vi "He magnet field realtime.vi"() -> ()   [LabVIEW 2016]
uses:
  <vilib>/rvi/interface/nirviReadWriteControl/nirviReadWriteControl.xnode
  <vilib>/rvi/interface/nirviOpenFPGA/nirviOpenFPGA.xnode
  HE Fpga/He magnet field fpga.vi
  <vilib>/Utility/error.llb/Error Cluster From Error Code.vi
  <vilib>/rvi/errors/niLvFpgaAdjustHostInterfaceError.vi
  NiFpgaLv.dll
  FPGA Bitfiles/Controlsoftware2_FPGATarget3_Hemagnetfieldfpg_5TwZ+QBV9Tk.lvbitx
  <vilib>/FPGAPlugInAG/cRIO-9074/niLvFpga_Open_cRIO-9074.vi
panel:
  out "He Quad B I":fxp<+/-,26,5> format="%.3g"
  in  "Ion gauge cluster control":T1
  in  "Tab Control":enum32{"Extra", "Controls"}(tab)
  out "Convectron 3":u8[](array[numeric])
  out "Ion gauge 4":u8[](array[numeric])
  out "Convectron 4":u8[](array[numeric])
  out "Ion gauge 5":u8[](array[numeric])
  out "Convectron 2":u8[](array[numeric])
  out "Ion gauge 2":u8[](array[numeric])
  out "Convectron 1":u8[](array[numeric])
  out "Ion gauge 1":u8[](array[numeric])
  out "He Quad B I":fxp<+/-,26,5> format="%.3g"
  out "He Quad B V":fxp<+/-,26,5> format="%.3g"
  out "He Quad A I":fxp<+/-,26,5> format="%.3g"
  out "He Quad A V":fxp<+/-,26,5> format="%.3g"
  out "Y-I":fxp<+/-,26,5> format="%.3g"
  out "Y-V":fxp<+/-,26,5> format="%.3g"
  out "Y+I":fxp<+/-,26,5> format="%.3g"
  out "Y+ V":fxp<+/-,26,5> format="%.3g"
  out "X-I":fxp<+/-,26,5> format="%.3g"
  out "X- V":fxp<+/-,26,5> format="%.3g"
  out "X+ I":fxp<+/-,26,5> format="%.3g"
  out "X+ V":fxp<+/-,26,5> format="%.3g"
  out "Y Steerer -":dbl
  out "Y Steerer +":dbl
  out "Y Steerer - 2":dbl
  out "Y Steerer + 2":dbl
  out "X Steerer -":dbl
  out "X Steerer +":dbl
  out "He Quad B":dbl
  out "He Quad A":dbl
  out "Y-I 2":fxp<+/-,26,5> format="%.3g"
  out "Y-V 2":fxp<+/-,26,5> format="%.3g"
  out "Y+I 2":fxp<+/-,26,5> format="%.3g"
  out "Y+ V  2":fxp<+/-,26,5> format="%.3g"
  out "Analyze IN?":bool
  out "Analyze Out?":bool
  out "Tank Exit FC":bool
  out "Analyze Image FC":bool
  out "Ion gauge cluser 2":T1
  out "Ion gauge Cluster 1":T1
  out "error out 3":errorcluster
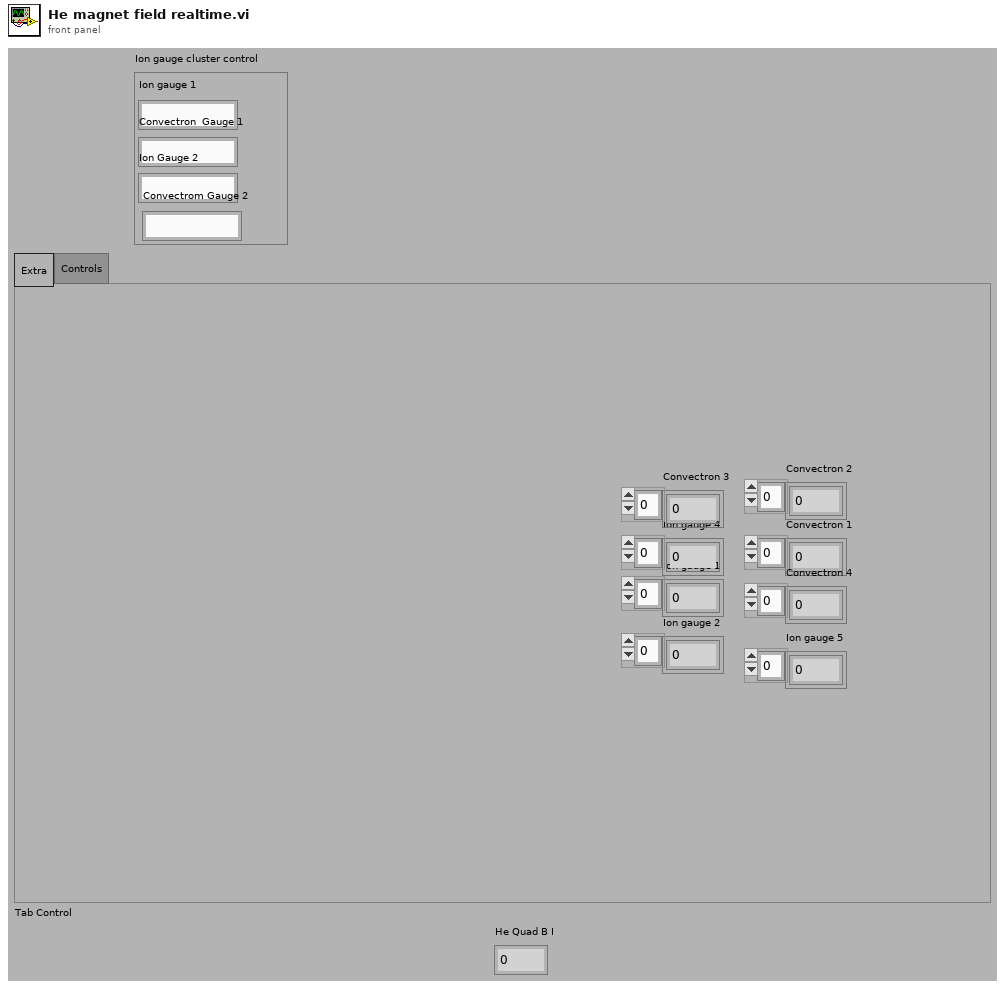
[diagram p1: front panel]
types:
  T1 = cluster{"Ion gauge 1":string, "Convectron  Gauge 1 ":string, "Ion Gauge 2":string, "Convectrom Gauge 2":string}
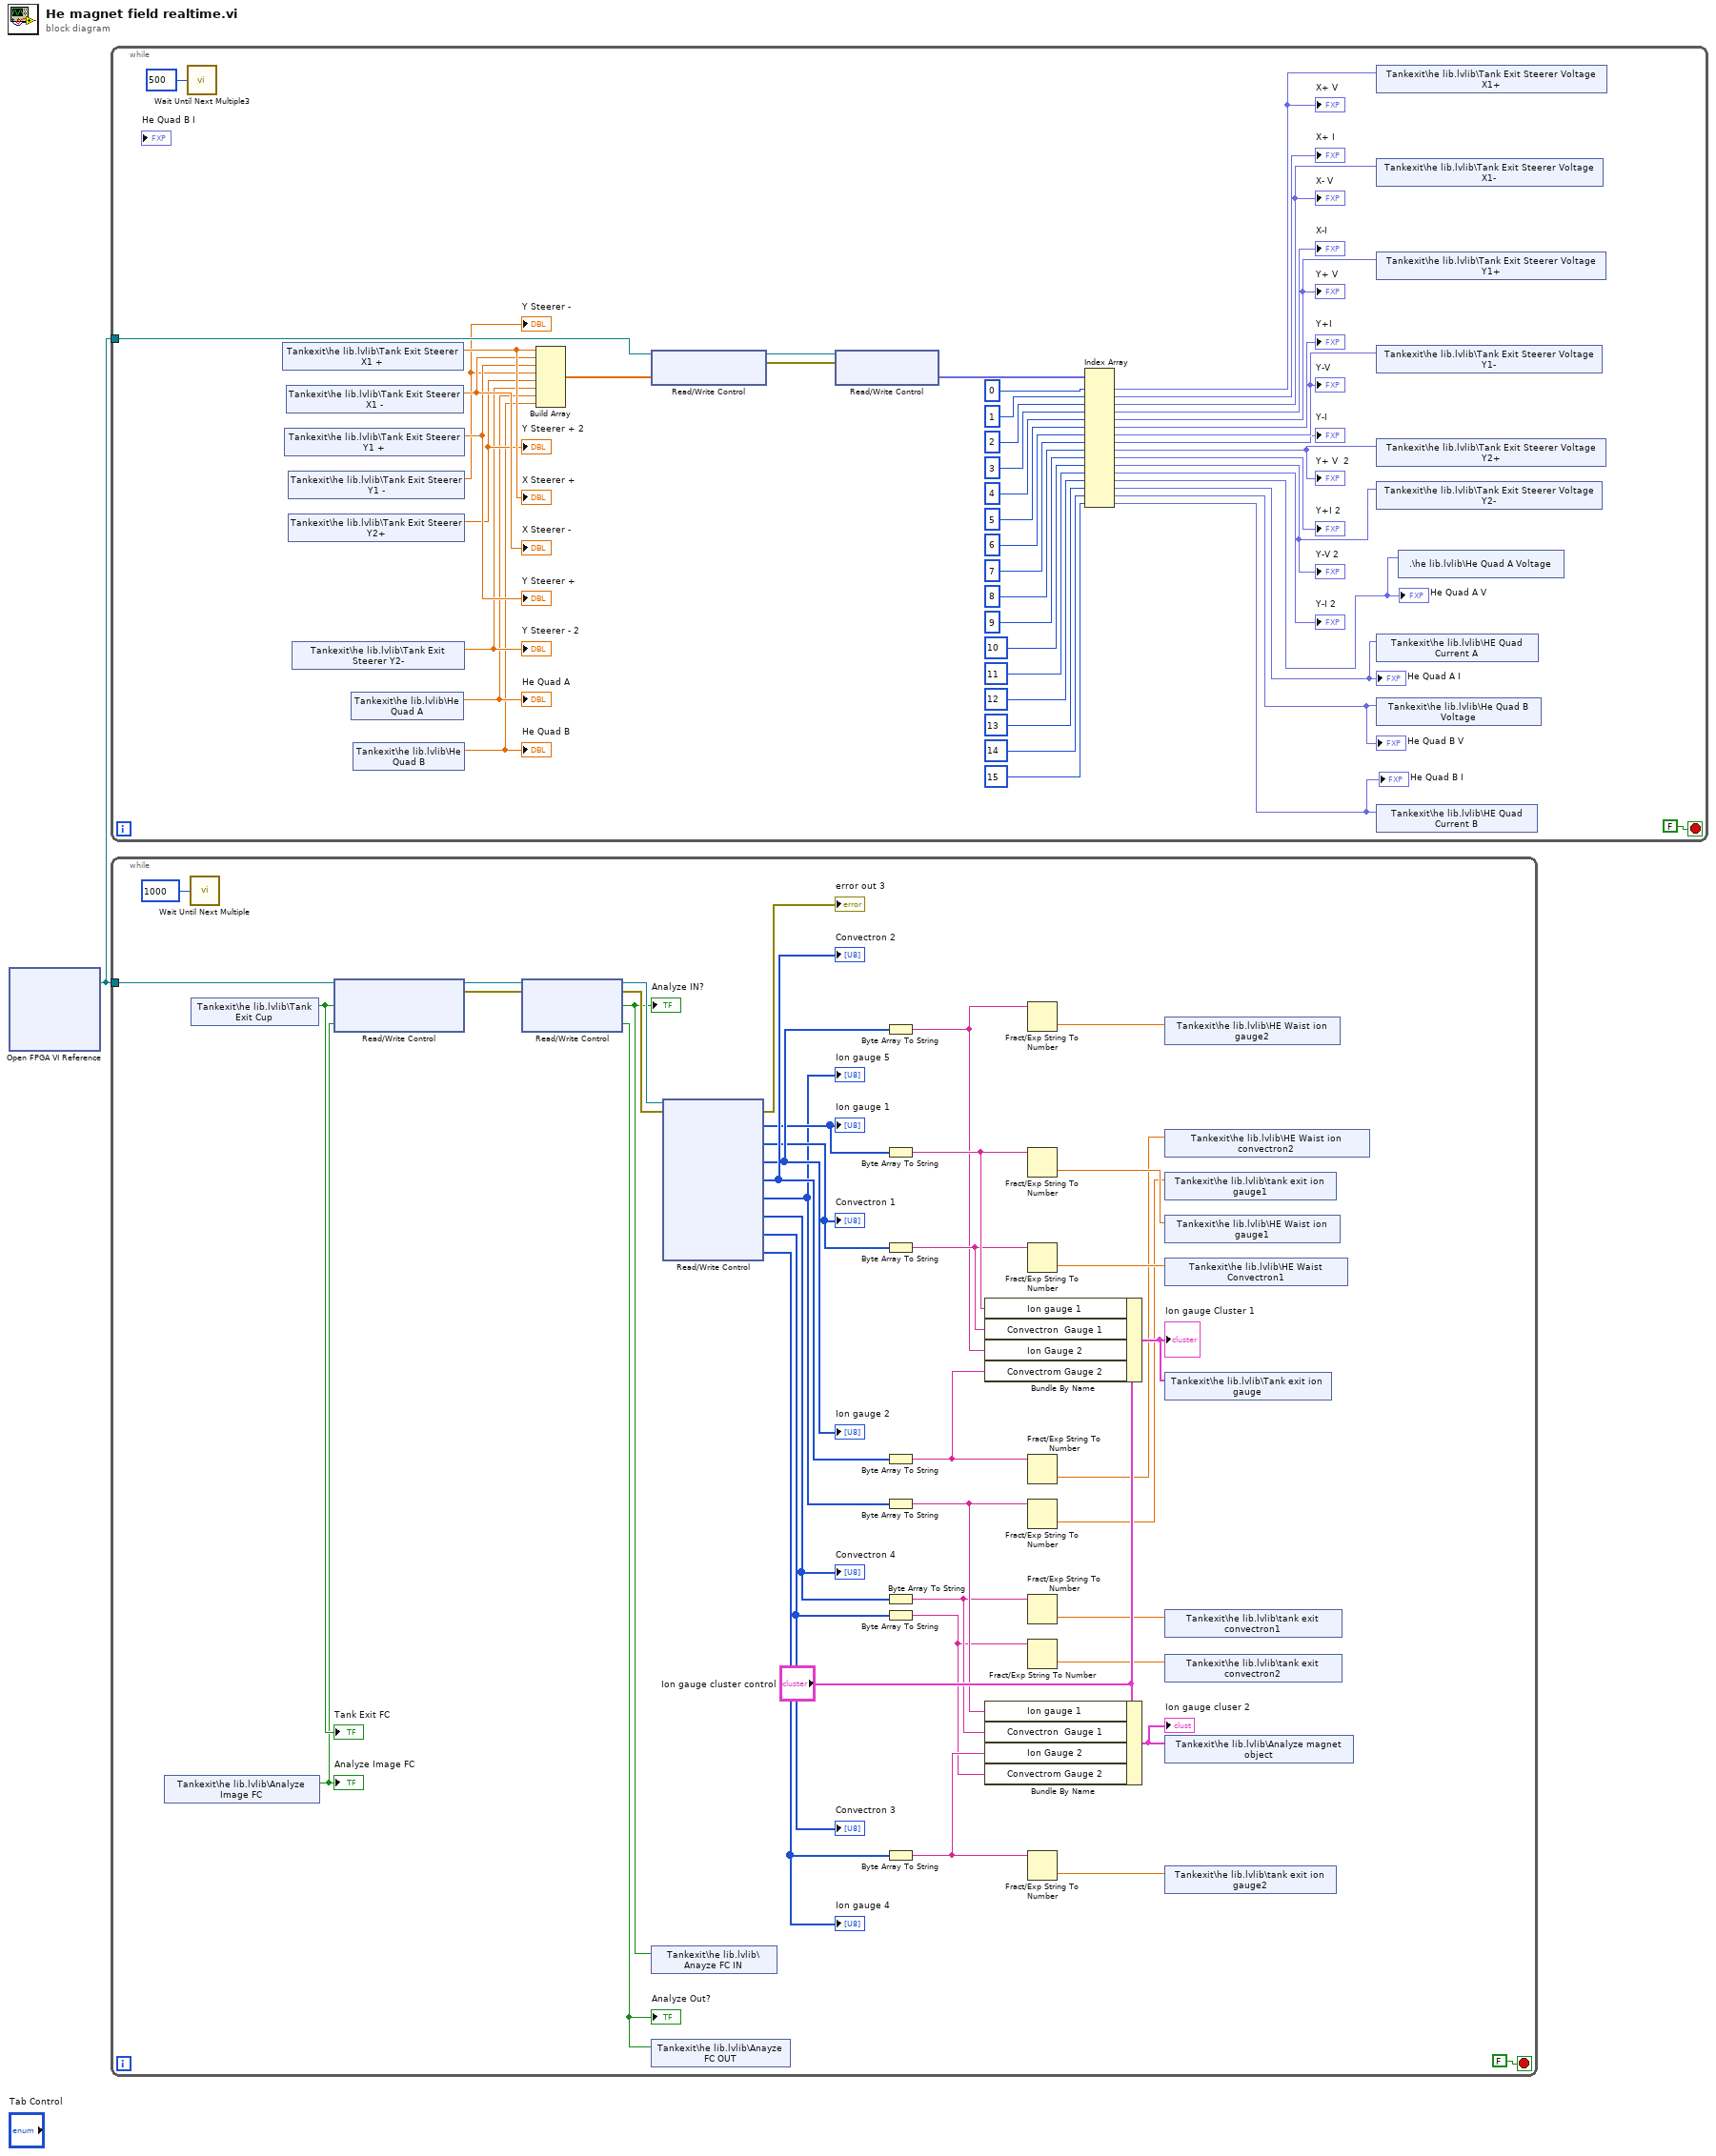
[diagram p0: block diagram]
diagram:
  n1 = xnode "Open FPGA VI Reference"() -> ("FPGA VI Reference Out"=w1:refnum<k20>)  [unwired: 2 in, 1 out]
  n2 = while {
    tunnel: w1 -> [w47]
    stop <- FALSE stop-if-true
    n3 = call "Wait Until Next Multiple3"("Count(mSec)"=u32 500 ("Count(uSec)")) -> ()  [unwired: 1 out]
    n4 = shared-variable "Tankexit\\he lib.lvlib\\Tank Exit Steerer X1 +"() -> (w25:dbl)  [unwired: 1 in, 1 out]
    "X Steerer +" <- w25
    n5 = shared-variable "Tankexit\\he lib.lvlib\\Tank Exit Steerer Y1 +"() -> (w23:dbl)  [unwired: 1 in, 1 out]
    "Y Steerer +" <- w23
    n6 = shared-variable "Tankexit\\he lib.lvlib\\Tank Exit Steerer X1 -"() -> (w24:dbl)  [unwired: 1 in, 1 out]
    "X Steerer -" <- w24
    n7 = shared-variable "Tankexit\\he lib.lvlib\\Tank Exit Steerer Y1 -"() -> (w22:dbl)  [unwired: 1 in, 1 out]
    "Y Steerer -" <- w22
    n8 = shared-variable "Tankexit\\he lib.lvlib\\Tank Exit Steerer Y2+"() -> (w21:dbl)  [unwired: 1 in, 1 out]
    "Y Steerer + 2" <- w21
    n9 = shared-variable "Tankexit\\he lib.lvlib\\Tank Exit Steerer Y2-"() -> (w20:dbl)  [unwired: 1 in, 1 out]
    "Y Steerer - 2" <- w20
    n10 = shared-variable "Tankexit\\he lib.lvlib\\He Quad A"() -> (w19:dbl)  [unwired: 1 in, 1 out]
    "He Quad A" <- w19
    n11 = shared-variable "Tankexit\\he lib.lvlib\\He Quad B"() -> (w18:dbl)  [unwired: 1 in, 1 out]
    "He Quad B" <- w18
    n12 = Build Array(w25, w24, w23, w22, w21, w20, w19, w18) -> (w48:dbl[])
    n13 = xnode "Read/Write Control"("FPGA VI Reference In"=w47, "Analog Output"=w48) -> ("FPGA VI Reference Out"=w34:refnum<k20>, "error out"=w30:errorcluster)  [unwired: 1 in]
    n14 = xnode "Read/Write Control"("FPGA VI Reference In"=w34, "error in"=w30) -> ("Analog input"=w33:fxp<+/-,26,5>[])  [unwired: 2 out]
    n15 = Index Array(array=w33, index #1=0 ("index"), index #2=1 ("index"), index #3=2 ("index"), index #4=3 ("index"), index #5=4 ("index"), index #6=5 ("index"), index #7=6 ("index"), index #8=7 ("index"), index #9=8 ("index"), index #10=9 ("index"), index #11=10 ("index"), index #12=11 ("index"), index #13=12 ("index"), index #14=13 ("index"), index #15=14 ("index"), index #16=15 ("index")) -> (element #1=w17:fxp<+/-,26,5>, element #2=→"X+ I":fxp<+/-,26,5>, element #3=w15:fxp<+/-,26,5>, element #4=→"X-I":fxp<+/-,26,5>, element #5=w13:fxp<+/-,26,5>, element #6=→"Y+I":fxp<+/-,26,5>, element #7=w11:fxp<+/-,26,5>, element #8=→"Y-I":fxp<+/-,26,5>, element #9=w9:fxp<+/-,26,5>, element #10=→"Y+I 2":fxp<+/-,26,5>, element #11=w6:fxp<+/-,26,5>, element #12=→"Y-I 2":fxp<+/-,26,5>, element #13=w3:fxp<+/-,26,5>, element #14=w4:fxp<+/-,26,5>, element #15=w5:fxp<+/-,26,5>, element #16=w2:fxp<+/-,26,5>)
    "X+ V" <- w17
    "X- V" <- w15
    "Y+ V" <- w13
    "Y-V" <- w11
    "He Quad A V" <- w3
    "He Quad A I" <- w4
    "He Quad B V" <- w5
    "Y+ V  2" <- w9
    "Y-V 2" <- w6
    "He Quad B I" <- w2
    n16 = shared-variable "Tankexit\\he lib.lvlib\\Tank Exit Steerer Voltage X1+"(w17) -> ()  [unwired: 1 in, 1 out]
    n17 = shared-variable "Tankexit\\he lib.lvlib\\Tank Exit Steerer Voltage X1-"(w15) -> ()  [unwired: 1 in, 1 out]
    n18 = shared-variable "Tankexit\\he lib.lvlib\\Tank Exit Steerer Voltage Y1+"(w13) -> ()  [unwired: 1 in, 1 out]
    n19 = shared-variable "Tankexit\\he lib.lvlib\\Tank Exit Steerer Voltage Y1-"(w11) -> ()  [unwired: 1 in, 1 out]
    n20 = shared-variable "Tankexit\\he lib.lvlib\\Tank Exit Steerer Voltage Y2+"(w9) -> ()  [unwired: 1 in, 1 out]
    n21 = shared-variable "Tankexit\\he lib.lvlib\\Tank Exit Steerer Voltage Y2-"(w6) -> ()  [unwired: 1 in, 1 out]
    n22 = shared-variable "Tankexit\\he lib.lvlib\\HE Quad Current A"(w4) -> ()  [unwired: 1 in, 1 out]
    n23 = shared-variable "Tankexit\\he lib.lvlib\\He Quad B Voltage"(w5) -> ()  [unwired: 1 in, 1 out]
    n24 = shared-variable "Tankexit\\he lib.lvlib\\HE Quad Current B"(w2) -> ()  [unwired: 1 in, 1 out]
    n25 = shared-variable ".\\he lib.lvlib\\He Quad A Voltage"(w3) -> ()  [unwired: 1 in, 1 out]
  }
  n26 = while {
    tunnel: w1 -> [w76]
    stop <- FALSE stop-if-true
    n27 = shared-variable "Tankexit\\he lib.lvlib\\Analyze Image FC"() -> (w70:bool)  [unwired: 1 in, 1 out]
    "Analyze Image FC" <- w70
    n28 = call "Wait Until Next Multiple"("Count(mSec)"=u32 1000 ("millisecond multiple")) -> ()  [unwired: 1 out]
    n29 = shared-variable "Tankexit\\he lib.lvlib\\Tank Exit Cup"() -> (w71:bool)  [unwired: 1 in, 1 out]
    "Tank Exit FC" <- w71
    n30 = xnode "Read/Write Control"("FPGA VI Reference In"=w76, "Tank Exit FC"=w71, "Analyze Image FC"=w70) -> ("FPGA VI Reference Out"=w75:refnum<k20>, "error out"=w74:errorcluster)  [unwired: 1 in]
    n31 = xnode "Read/Write Control"("FPGA VI Reference In"=w75, "error in"=w74) -> ("FPGA VI Reference Out"=w72:refnum<k20>, "error out"=w73:errorcluster, "Analyze IN?"=w69:bool, "Analyze Out?"=w68:bool)
    "Analyze IN?" <- w69
    "Analyze Out?" <- w68
    n32 = shared-variable "Tankexit\\he lib.lvlib\\Anayze FC IN"(w69) -> ()  [unwired: 1 in, 1 out]
    n33 = shared-variable "Tankexit\\he lib.lvlib\\Anayze FC OUT"(w68) -> ()  [unwired: 1 in, 1 out]
    n34 = xnode "Read/Write Control"("FPGA VI Reference In"=w72, "error in"=w73) -> ("error out"=→"error out 3":errorcluster, "Ion gauge 1"=w84:u8[], "Convectron 1"=w85:u8[], "Ion gauge 2"=w86:u8[], "Convectron 2"=w87:u8[], "Ion gauge 3"=w81:u8[], "Convectron 3"=w80:u8[], "Convectron 4"=w78:u8[], "Ion gauge 4"=w79:u8[])  [unwired: 1 out]
    "Ion gauge 1" <- w84
    "Convectron 1" <- w85
    "Ion gauge 2" <- w86
    "Convectron 2" <- w87
    "Ion gauge 5" <- w81
    "Convectron 4" <- w80
    "Ion gauge 4" <- w79
    "Convectron 3" <- w78
    n35 = Byte Array To String(unsigned byte array=w86) -> (string=w58:string)
    n36 = Byte Array To String(unsigned byte array=w84) -> (string=w60:string)
    n37 = Byte Array To String(unsigned byte array=w85) -> (string=w59:string)
    n38 = Byte Array To String(unsigned byte array=w87) -> (string=w57:string)
    n39 = Byte Array To String(unsigned byte array=w81) -> (string=w64:string)
    n40 = Byte Array To String(unsigned byte array=w80) -> (string=w63:string)
    n41 = Byte Array To String(unsigned byte array=w78) -> (string=w61:string)
    n42 = Byte Array To String(unsigned byte array=w79) -> (string=w62:string)
    n43 = Bundle By Name(cluster="Ion gauge cluster control", "Ion gauge 1"=w60, "Convectron  Gauge 1"=w59, "Ion Gauge 2"=w58, "Convectrom Gauge 2"=w57) -> (w66:T1)
    "Ion gauge Cluster 1" <- w66
    n44 = Bundle By Name(cluster="Ion gauge cluster control", "Ion gauge 1"=w64, "Convectron  Gauge 1"=w63, "Ion Gauge 2"=w62, "Convectrom Gauge 2"=w61) -> (w67:T1)
    "Ion gauge cluser 2" <- w67
    n45 = Fract/Exp String To Number(string=w58) -> (number=w54:dbl)  [unwired: 3 in, 1 out]
    n46 = Fract/Exp String To Number(string=w60) -> (number=w56:dbl)  [unwired: 3 in, 1 out]
    n47 = Fract/Exp String To Number(string=w59) -> (number=w55:dbl)  [unwired: 3 in, 1 out]
    n48 = Fract/Exp String To Number(string=w57) -> (number=w53:dbl)  [unwired: 3 in, 1 out]
    n49 = Fract/Exp String To Number(string=w64) -> (number=w52:dbl)  [unwired: 3 in, 1 out]
    n50 = Fract/Exp String To Number(string=w63) -> (number=w50:dbl)  [unwired: 3 in, 1 out]
    n51 = Fract/Exp String To Number(string=w61) -> (number=w49:dbl)  [unwired: 3 in, 1 out]
    n52 = Fract/Exp String To Number(string=w62) -> (number=w51:dbl)  [unwired: 3 in, 1 out]
    n53 = shared-variable "Tankexit\\he lib.lvlib\\HE Waist ion gauge2"(w54) -> ()  [unwired: 1 in, 1 out]
    n54 = shared-variable "Tankexit\\he lib.lvlib\\HE Waist ion convectron2"(w53) -> ()  [unwired: 1 in, 1 out]
    n55 = shared-variable "Tankexit\\he lib.lvlib\\tank exit ion gauge1"(w52) -> ()  [unwired: 1 in, 1 out]
    n56 = shared-variable "Tankexit\\he lib.lvlib\\HE Waist ion gauge1"(w56) -> ()  [unwired: 1 in, 1 out]
    n57 = shared-variable "Tankexit\\he lib.lvlib\\HE Waist Convectron1"(w55) -> ()  [unwired: 1 in, 1 out]
    n58 = shared-variable "Tankexit\\he lib.lvlib\\Tank exit ion gauge"(w66) -> ()  [unwired: 1 in, 1 out]
    n59 = shared-variable "Tankexit\\he lib.lvlib\\tank exit convectron1"(w50) -> ()  [unwired: 1 in, 1 out]
    n60 = shared-variable "Tankexit\\he lib.lvlib\\tank exit convectron2"(w49) -> ()  [unwired: 1 in, 1 out]
    n61 = shared-variable "Tankexit\\he lib.lvlib\\Analyze magnet object"(w67) -> ()  [unwired: 1 in, 1 out]
    n62 = shared-variable "Tankexit\\he lib.lvlib\\tank exit ion gauge2"(w51) -> ()  [unwired: 1 in, 1 out]
  }
